vi "MANUAL_CONTROL.vi"(11 "Payload":T1) -> (3 "MAVLink Message":u8[](array[numeric]))   [LabVIEW 2014]
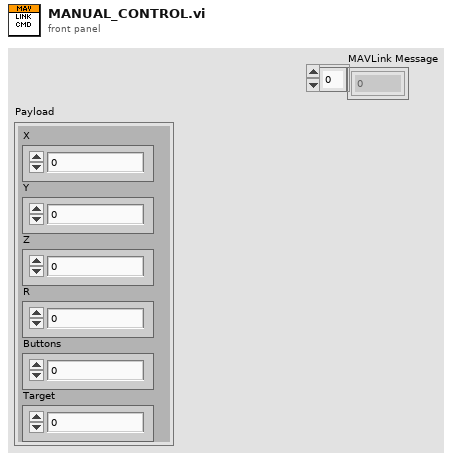
[diagram p1: front panel]
types:
  T1 = cluster{"X":i16, "Y":i16, "Z":i16, "R":i16, "Buttons":u16, "Target":u8}
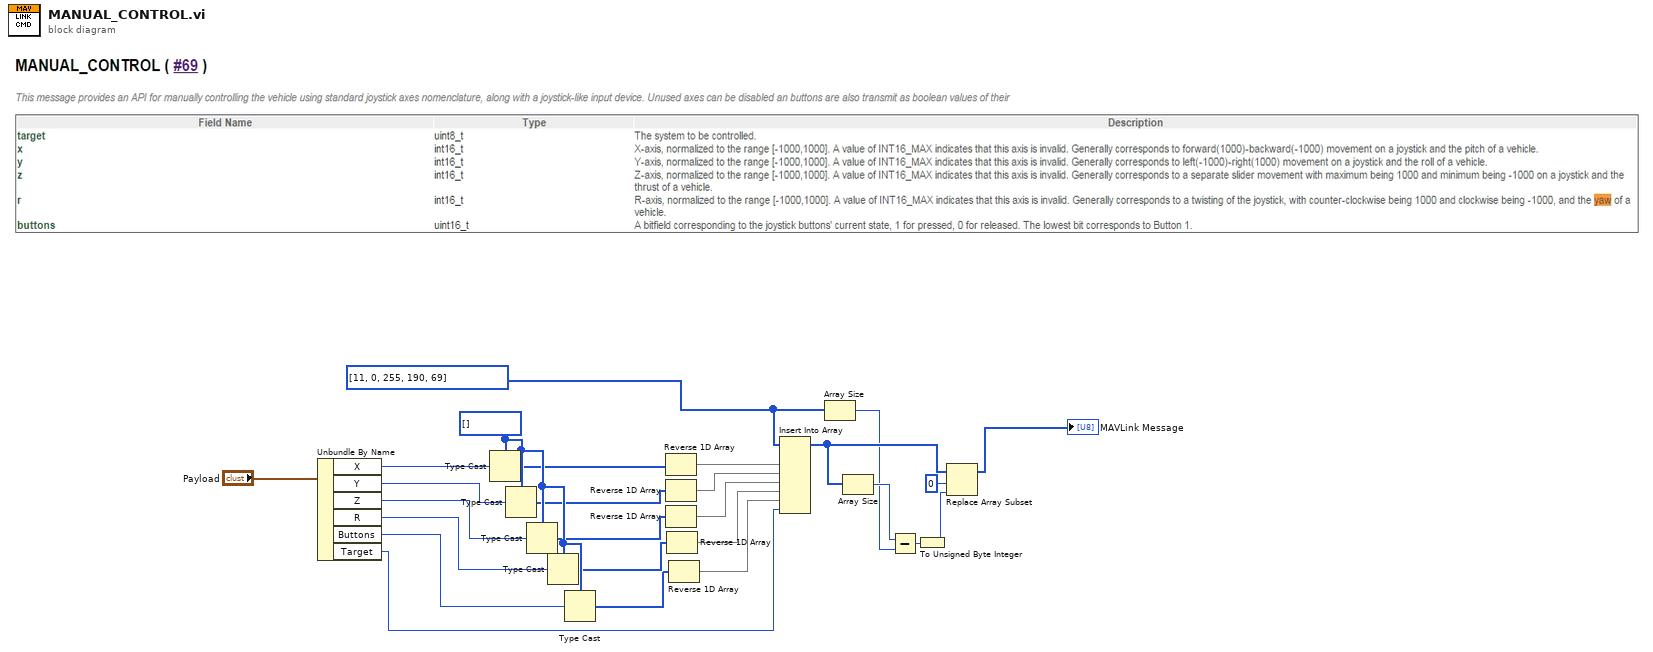
[diagram p0: block diagram]
diagram:
  w21 = u8[] []
  w3 = u8[] [11, 0, 255, 190, 69]
  n1 = Unbundle By Name("Payload") -> ("X"=w20:i16, "Y"=w19:i16, "Z"=w18:i16, "R"=w17:i16, "Buttons"=w16:u16, "Target"=w5:u8)
  n2 = Type Cast(type=w21, x=w20) -> (*(type *) &x=w15:u8[])
  n3 = Type Cast(type=w21, x=w19) -> (*(type *) &x=w14:u8[])
  n4 = Type Cast(type=w21, x=w18) -> (*(type *) &x=w13:u8[])
  n5 = Type Cast(type=w21, x=w17) -> (*(type *) &x=w12:u8[])
  n6 = Type Cast(type=w21, x=w16) -> (*(type *) &x=w11:u8[])
  n7 = Reverse 1D Array(array=w15) -> (reversed array=w10:u8[])
  n8 = Reverse 1D Array(array=w14) -> (reversed array=w9:u8[])
  n9 = Reverse 1D Array(array=w13) -> (reversed array=w8:u8[])
  n10 = Reverse 1D Array(array=w12) -> (reversed array=w7:u8[])
  n11 = Reverse 1D Array(array=w11) -> (reversed array=w6:u8[])
  n12 = Insert Into Array(array=w3, new element #1=w10, new element #2=w9, new element #3=w8, new element #4=w7, new element #5=w6, new element #6=w5) -> (w23:u8[])  [unwired: 1 in]
  n13 = Array Size(array=w3) -> (size(s)=w2:i32)
  n14 = Array Size(array=w23) -> (size(s)=w4:i32)
  n15 = Subtract(x=w4, y=w2) -> (x-y=w1:i32)
  n16 = To Unsigned Byte Integer(number=w1) -> (unsigned 8bit integer=w22:u8)
  n17 = Replace Array Subset(array=w23, new element=w22, index=0) -> (→"MAVLink Message":u8[])
